vi "solar_type Set Items (Types).vi"(6 "ArrayDelimiters (1D,2D)":string[](array[string]), 7 "Cluster Name (\"\")":string, 8 "error in (no error)":errorcluster, 9 "Values (ASCII)":string[](array[string]), 10 "Names (\"\")":string[](array[string]), 11 "Types":T1[](array[typedef])) -> (0 "error out":errorcluster, 3 "Variant out":variant)   [LabVIEW 2018]
doc: "This VI sets the variant value. This retains the attributes and type string."
uses:
  <vilib>/Utility/Data Type/NI_Data Type.lvlib
  solar_type Item Type.ctl
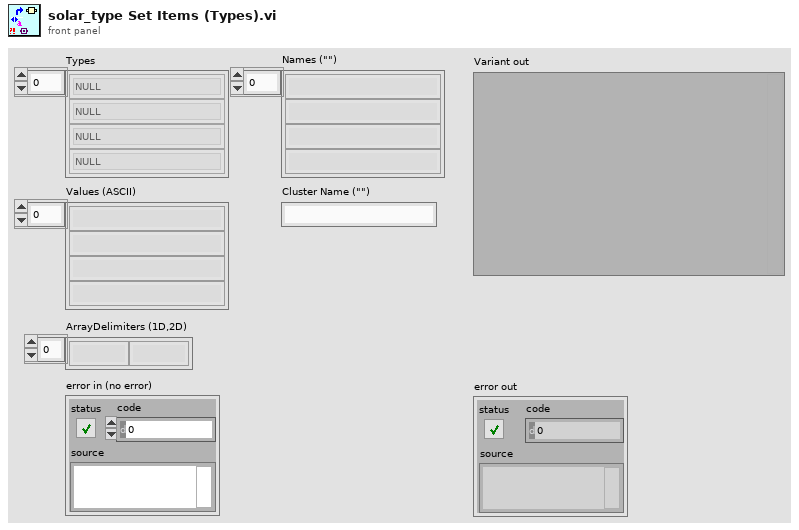
[diagram p1: front panel]
types:
  T1 = typedef "solar_type Item Type.ctl" = enum16{"NULL", "UNKNOWN", "CLUSTER", "I8", "I16", "I32", "I64", "U8", "U16", "U32", "U64", "U8_ENUM", "U16_ENUM", "U32_ENUM", "SGL", "DBL", "BOOLEAN", "STRING", "PATH", "VISA", "TAG", "TIME", "I8_1D", "I16_1D", "I32_1D", "I64_1D", "U8_1D", "U16_1D", "U32_1D", "U64_1D", "U8_ENUM_1D", "U16_ENUM_1D", "U32_ENUM_1D", "SGL_1D", "DBL_1D", "BOOLEAN_1D", "STRING_1D", "PATH_1D", "VISA_1D", "TAG_1D", "TIME_1D", "I8_2D", "I16_2D", "I32_2D", "I64_2D", "U8_2D", "U16_2D", "U32_2D", "U64_2D", "U8_ENUM_2D", "U16_ENUM_2D", "U32_ENUM_2D", "SGL_2D", "DBL_2D", "BOOLEAN_2D", "STRING_2D", "PATH_2D", "VISA_2D", "TAG_2D", "TIME_2D"}
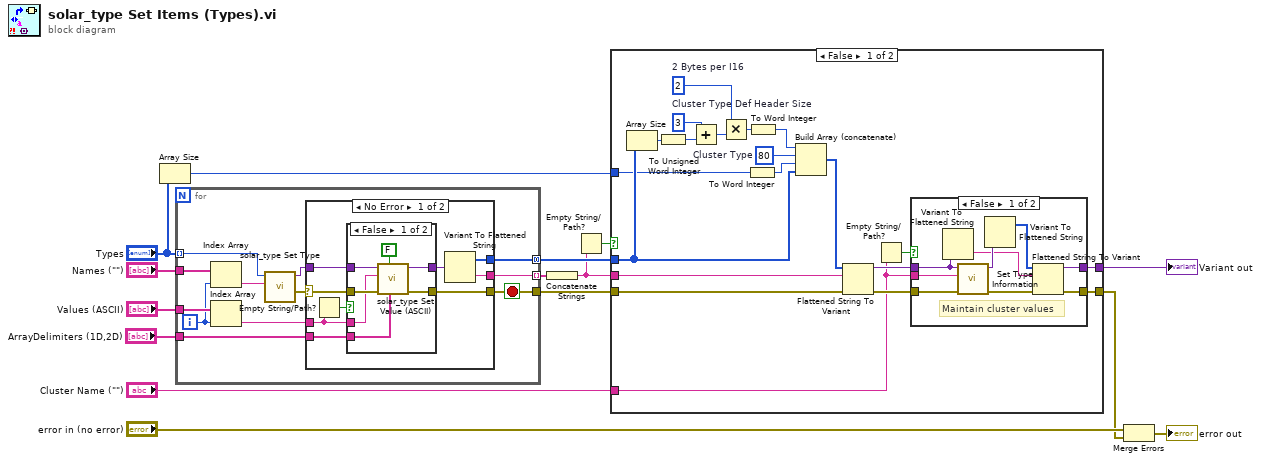
[diagram p0: block diagram]
diagram:
  n1 = Array Size(array="Types") -> (size(s)=w8:i32)
  n2 = for {
    tunnel: "Names (\"\")" -> [w27]
    tunnel: "Types" -> [w24] mode=indexing
    tunnel: [w16] -> w11 mode=concatenating
    tunnel: [w21] -> w10
    tunnel: [w18] -> w12 mode=indexing
    tunnel: "Values (ASCII)" -> [w23]
    tunnel: "ArrayDelimiters (1D,2D)" -> [w17]
    i -> [w20]
    stop <- w21 stop-if-true
    n3 = Index Array(array=w27, index=w20) -> (element=w26:string)
    n4 = Index Array(array=w23, index=w20) -> (element=w19:string)
    n5 = call "solar_type Set Type.vi"("Name"=w26, "Type"=w24) -> ("error out"=w22:errorcluster, "Variant"=w25:variant)  [unwired: 6 in]
    n6 = case shown="No Error" w22 {
      selector: w22 -> [w36 w46]
      tunnel: w25 -> [w31 _]
      tunnel: [w35 w46] -> w21
      tunnel: w19 -> [w34 _]
      tunnel: [w29 _] -> w18
      tunnel: w17 -> [w32 _]
      tunnel: [w28 _] -> w16
      frame No Error {
        n7 = Empty String/Path?(string/path=w34) -> (empty?=w33:bool)
        n8 = case shown="False" w33 {
          tunnel: w36 -> [w43 w45]
          tunnel: [w42 w45] -> w35
          tunnel: w34 -> [w39 _]
          tunnel: w31 -> [w38 w44]
          tunnel: [w41 w44] -> w30
          tunnel: w32 -> [w40 _]
          frame False {
            n9 = call "solar_type Set Value (ASCII).vi"("ArrayDelimiters (1D,2D)"=w40, "Keep Attributes? (F)"=FALSE, "error in (no error)"=w43, "Value (ASCII)"=w39, "Variant"=w38) -> ("error out"=w42:errorcluster, "Variant out"=w41:variant)  [unwired: 4 in, 1 out]
          }
          frame True {
          }
        }
        n10 = Variant To Flattened String(Variant=w30) -> (data string=w29:string, 1:w28:i16[])
      }
      frame Error {
      }
    }
  }
  n11 = Concatenate Strings(w12) -> (w2:string)
  n12 = Empty String/Path?(string/path=w2) -> (empty?=w1:bool)
  n13 = case shown="False" w1 {
    tunnel: w11 -> [w57 _]
    tunnel: w10 -> [w56 w78]
    tunnel: w8 -> [w54 _]
    tunnel: [w51 _] -> w6
    tunnel: [w49 w78] -> w5
    tunnel: "Cluster Name (\"\")" -> [w48 _]
    tunnel: w2 -> [w47 _]
    frame False {
      w58 = i16 80  # Cluster Type
      w61 = u16 2  # 2 Bytes per I16
      w63 = u16 3  # Cluster Type Def Header Size
      n14 = Array Size(array=w57) -> (size(s)=w66:i32)
      n15 = To Unsigned Word Integer(number=w66) -> (unsigned 16bit integer=w60:u16)
      n16 = Add(x=w63, y=w60) -> (x+y=w62:u16)
      n17 = Multiply(x=w61, y=w62) -> (x*y=w59:u16)
      n18 = To Word Integer(number=w54) -> (16bit integer=w64:i16)
      n19 = To Word Integer(number=w59) -> (16bit integer=w65:i16)
      n20 = Build Array (concatenate)(w65, w58, w64, w57) -> (w55:i16[])
      n21 = Flattened String To Variant(4:w56, 6:w47, 7:w55) -> (0:w50:errorcluster, 3:w52:variant)
      n22 = Empty String/Path?(string/path=w48) -> (empty?=w53:bool)
      n23 = case shown="False" w53 {
        tunnel: [w69 w76] -> w49
        tunnel: w50 -> [w74 w76]
        tunnel: w48 -> [w75 _]
        tunnel: w52 -> [w73 w77]
        tunnel: [w68 w77] -> w51
        frame False {
          # "Maintain cluster values"
          n24 = Variant To Flattened String(Variant=w73) -> (data string=w67:string)  [unwired: 1 out]
          n25 = call <vilib>:"Set Type Information.vi"("error in (no error)"=w74, "Name"=w75, "Variant in"=w73) -> ("error out"=w72:errorcluster, "Variant out"=w71:variant)  [unwired: 7 in]
          n26 = Variant To Flattened String(Variant=w71) -> (1:w70:i16[])  [unwired: 1 out]
          n27 = Flattened String To Variant(4:w72, 6:w67, 7:w70) -> (0:w69:errorcluster, 3:w68:variant)
        }
        frame True {
        }
      }
    }
    frame True {
    }
  }
  "Variant out" <- w6
  n28 = Merge Errors("error in (no error)", w5) -> (→"error out":errorcluster)
